vi "GSI-HVSwitch2.i attribute.vi"(0 "VI Refnum":refnum<vi>, 2 "CLASS.i attribute":T1={"SDEX VISA Cluster"={"VISA resource name"="", "HEX address"=0, "VISA Timeout Value (1000 ms)"=1000, "Lock Timeout (1000 ms)"=1000, "semaphore"=refnum, "Baud rate"=0, "revision"=enum."unknown", "deviceInfo"=""}, "SetVoltage SW0"=0.0, "SetVoltage SW1"=0.0, "ActTempAmp"=0.0, "ActTempPS1"=0.0, "ActTempPS2"=0.0, "mode"=enum."unknown", "interfaceInitialized"=FALSE, "serviceIDs"={"nomVoltage0ID"=0, "nomVoltage1ID"=0, "actTempAmpID"=0, "actTempPS1ID"=0, "actTempPS2ID"=0, "modeID"=0}, "usedChannels"=0} {"SDEX VISA Cluster"."HEX address" format="%.0x"}, 3 "Action":T6(ring), 5 "error in (no error)":errorcluster) -> (14 "VI Refnum out":refnum<vi>, 16 "CLASS.i attribute out":T1={"SDEX VISA Cluster"={"VISA resource name"="", "HEX address"=0, "VISA Timeout Value (1000 ms)"=1000, "Lock Timeout (1000 ms)"=1000, "semaphore"=refnum, "Baud rate"=0, "revision"=enum."unknown", "deviceInfo"=""}, "SetVoltage SW0"=0.0, "SetVoltage SW1"=0.0, "ActTempAmp"=0.0, "ActTempPS1"=0.0, "ActTempPS2"=0.0, "mode"=enum."unknown", "interfaceInitialized"=FALSE, "serviceIDs"={"nomVoltage0ID"=0, "nomVoltage1ID"=0, "actTempAmpID"=0, "actTempPS1ID"=0, "actTempPS2ID"=0, "modeID"=0}, "usedChannels"=0} {"SDEX VISA Cluster"."HEX address" format="%.0x"}, 19 "error out":errorcluster)   [LabVIEW 2014, in "GSI-HVSwitch2.lvlib"]
doc: "This is a so-called functional global variable. It manages the access to a global variable in a thread-safe way. \n\nHere the attribute data of all instances of THIS class are stored. This is done for performance reasons.\n\nLicense Agreement for this software:\n\nCopyright (C)\nGesellschaft für Schwerionenforschung, GSI\nPlanckstr. 1\n64291 Darmstadt\nGermany\n\nContact: D.Beck@gsi.de \n\nThis program is free software; you can redistribute it and/or modify it under the terms of the GNU General Public License as published by the Free Software Foundation; either version 2 of the license, or (at your option) any later version.\n\nThis program is distributed in the hope that it will be useful, but WITHOUT ANY WARRANTY; without even the implied warranty of MERCHANTABILITY or FITNESS FOR A PARTICULAR PURPOSE. See the GNU General License for more details (http://www.gnu.org).\n\nGesellschaft für Schwerionenforschung, GSI\nPlanckstr. 1, 64291 Darmstadt, Germany\nFor all questions and ideas contact: M.Richter@gsi.de, H.Brand@gsi.de or D.Beck@gsi.de.\nLast update: 17-JUN-2004"
uses:
  GSI-HVSwitch2.lvlib
  GSI-HVSwitch2.i attribute.ctl
  instr.lib/SDEX/SDEX.VISA Control.ctl
  instr.lib/SDEX/SDEX.revisionType.ctl
  GSI-HVSwitch2.mode.ctl
  CS_Core/CSSystem/CoreDefs/CoreDefs.error_type.ctl
  CS_Core/CSSystem/CoreLib/CoreLib.lvlib
  instr.lib/SDEX/SDEXDriver.lvlib
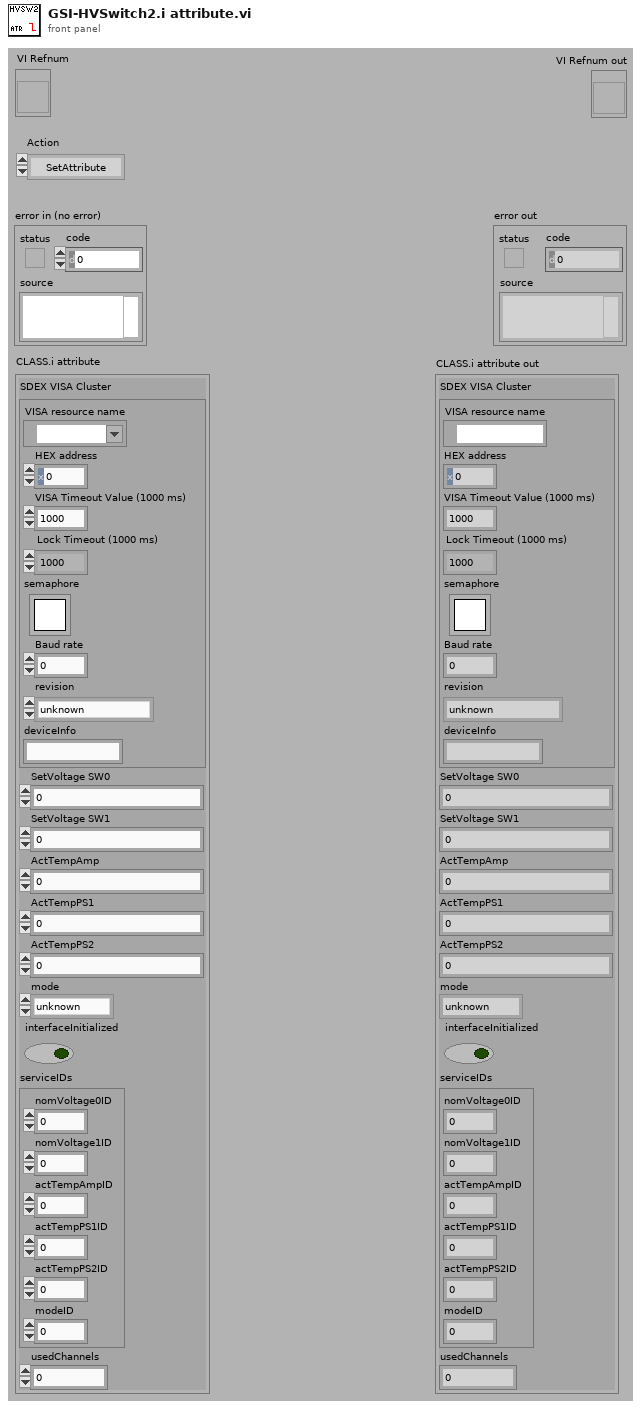
[diagram p1: front panel]
types:
  T1 = typedef "GSI-HVSwitch2.lvlib/GSI-HVSwitch2.i attribute.ctl" = cluster{"SDEX VISA Cluster":T2, "SetVoltage SW0":dbl, "SetVoltage SW1":dbl, "ActTempAmp":dbl, "ActTempPS1":dbl, "ActTempPS2":dbl, "mode":T5, "interfaceInitialized":bool, "serviceIDs":cluster{"nomVoltage0ID":i32, "nomVoltage1ID":i32, "actTempAmpID":i32, "actTempPS1ID":i32, "actTempPS2ID":i32, "modeID":i32}, "usedChannels":i32}
  T2 = typedef "SDEXDriver.lvlib/SDEX.VISA Control.ctl" = cluster{"VISA resource name":refnum<visa-resource-name>, "HEX address":u16, "VISA Timeout Value (1000 ms)":u32, "Lock Timeout (1000 ms)":u32, "semaphore":T3, "Baud rate":u32, "revision":T4, "deviceInfo":string}
  T3 = typedef "Semaphore RefNum" = refnum<k1>
  T4 = typedef "SDEXDriver.lvlib/SDEX.revisionType.ctl" = enum16{"unknown", "hvamp3", "hvswi1", "htrp0", "WDG0"}
  T5 = typedef "GSI-HVSwitch2.lvlib/GSI-HVSwitch2.mode.ctl" = enum16{"unknown", "switch", "stepper"}
  T6 = enum16{"SetAttribute", "GetAttribute", "CreateAttribute", "DestroyAttribute", "DestroyAllAtributes"}
  T7 = typedef "CoreDefs.error_type.ctl" = enum16{"no error", "can't load process", "can't unload process", "process does not exist", "can't install process", "can't remove process", "unknown function", "time out", "can't execute function", "duplicate queue name", "super not found", "caller queue invalid", "can't ping process", "unknown error", "VISA Error", "VISA timeout", "GPIB timeout", "GPIB error", "communication error", "data type mismatch", "can't read data from OPC server", "can't write data to OPC server", "OET error", "function not implemented", "process already exists", "invalid Shared Variable name", "error writing Shared Variable", "error reading Shared Variable", "invalid client name", "corrupt database", "unknown class", "call not authorized", "parameter out of range", "OET timeout: can't get data to modify", "invalid queue name", "requested operation incompatible with current state", "event undefined", "event disabled", "state undefined", "caller is not a friend", "EventBuilder: bad eventID", "EventBuilder: no DAQ devices", "a thread must not stop itself", "UNUSED ELEMENT4", "DiscArchiver: eventData incomplete", "DiscArchiver: eventData does not belong to run", "DiscArchiver: can't open file", "DiscArchiver: can't write to file", "DiscArchiver: available disc space low", "can't acquire semaphore", "error reading data from database", "notifier object is not existing", "can't register process", "can't unregister process", "illegal event type", "object disabled", "object already exists", "can't change state", "Instrument not found", "no connection to remote node", "invalid reference", "N/A", "UNUSED ELEMENT 1", "element not found", "illegal TCP/IP connection detected", "object does not exist", "invalid access ID", "unknown CS system", "invalid privilige", "unsupported data type", "unsupported server type", "IO server already exists", "Shared Variable already exists"}
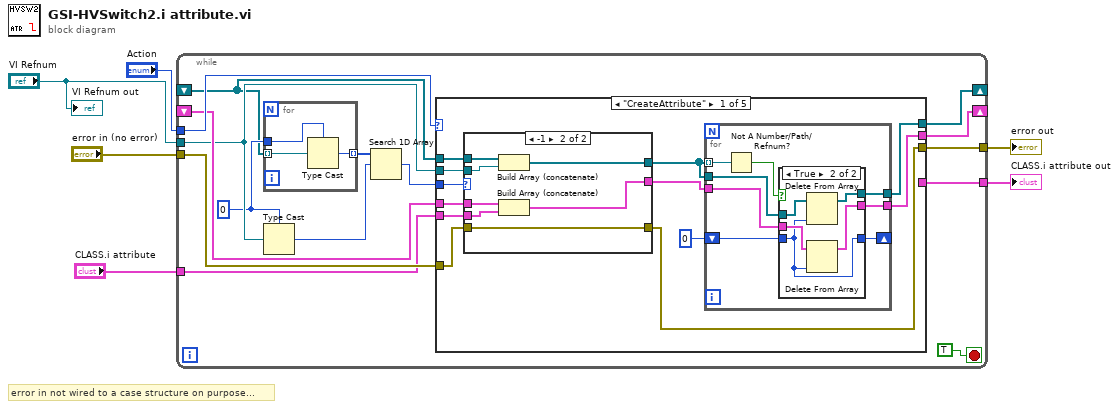
[diagram p0: block diagram]
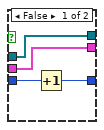
[diagram p2: hidden frame]
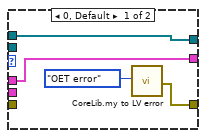
[diagram p3: hidden frame]
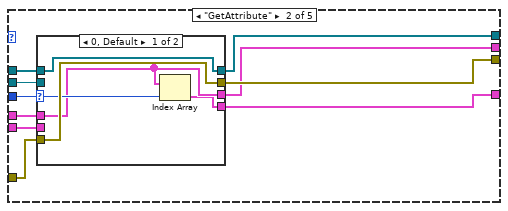
[diagram p4: hidden frame]
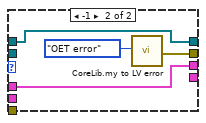
[diagram p5: hidden frame]
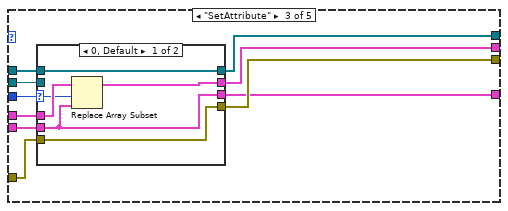
[diagram p6: hidden frame]
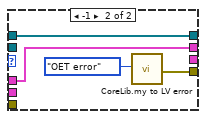
[diagram p7: hidden frame]
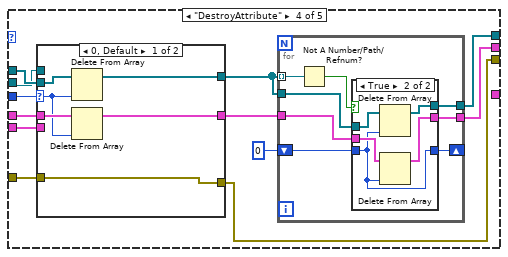
[diagram p8: hidden frame]
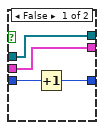
[diagram p9: hidden frame]
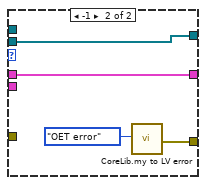
[diagram p10: hidden frame]
diagram:
  # "error in not wired to a case structure on purpose..."
  n1 = while {
    shift-right: [w15] -> _
    shift-left: _ -> [w16]
    tunnel: "Action" -> [w20]
    shift-right: [w17] -> _
    shift-left: _ -> [w7]
    tunnel: "error in (no error)" -> [w19]
    tunnel: [w18] -> w4
    tunnel: "CLASS.i attribute" -> [w14]
    tunnel: [w12] -> w2
    tunnel: "VI Refnum" -> [w10]
    stop <- TRUE stop-if-true
    w9 = 0
    n2 = for {
      tunnel: w9 -> [w24]
      tunnel: [w23] -> w8 mode=indexing
      tunnel: w7 -> [w22] mode=indexing
      n3 = Type Cast(type=w24, x=w22) -> (*(type *) &x=w23:i32)
    }
    n4 = Type Cast(type=w9, x=w10) -> (*(type *) &x=w11:i32)
    n5 = Search 1D Array(1D array=w8, element=w11) -> (index of element=w13:i32)  [unwired: 1 in]
    n6 = case shown="\"CreateAttribute\"" w20 {
      tunnel: w7 -> [w34 w72 w91 w113 _]
      tunnel: w10 -> [w33 w70 w89 w112 _]
      tunnel: w19 -> [w36 w74 w93 w115 w143]
      tunnel: [w35 w73 w92 w114 w143] -> w18
      tunnel: [w28 w71 w90 w107 _] -> w17
      tunnel: w16 -> [w32 w69 w88 w111 _]
      tunnel: [w27 w68 w87 w106 _] -> w15
      tunnel: w14 -> [w31 w67 w86 w110 _]
      tunnel: w13 -> [w30 w66 w85 w109 _]
      tunnel: [_ w65 w84 _ _] -> w12
      frame "CreateAttribute" {
        n7 = case shown="-1" w30 {
          tunnel: w36 -> [_ w64]
          tunnel: [w56 w64] -> w35
          tunnel: w34 -> [w55 w63]
          tunnel: [w55 w62] -> w25
          tunnel: w33 -> [_ w61]
          tunnel: w32 -> [w54 w60]
          tunnel: [w54 w59] -> w26
          tunnel: w31 -> [_ w58]
          frame 0, Default {
            n8 = call "CoreLib.my to LV error.vi"("ErrorTypes"=CoreDefs.error_type."OET error") -> ("myErrorCluster"=w56:errorcluster)  [unwired: 17 in, 1 out]
          }
          frame -1 {
            n9 = Build Array (concatenate)(w63, w61) -> (w62:refnum<vi>[])
            n10 = Build Array (concatenate)(w60, w58) -> (w59:T1[])
          }
        }
        n11 = for {
          tunnel: w25 -> [w41]
          tunnel: [w40] -> w28
          tunnel: [w44] -> w27
          tunnel: w26 -> [w43]
          tunnel: w25 -> [w39] mode=indexing
          shift-right: [w38] -> _
          shift-left: 0 -> [w37]
          n12 = Not A Number/Path/Refnum?(number/path/refnum=w39) -> (NaN/Path/Refnum?=w42:bool)
          n13 = case shown="True" w42 {
            tunnel: [w48 w53] -> w44
            tunnel: w43 -> [w48 w52]
            tunnel: [w47 w50] -> w40
            tunnel: w41 -> [w47 w51]
            tunnel: w37 -> [w46 w49]
            tunnel: [w45 w49] -> w38
            frame False {
              n14 = Increment(x=w46) -> (x+1=w45:i32)
            }
            frame True {
              n15 = Delete From Array(array=w51, index=w49) -> (array with subset deleted=w50:refnum<vi>[])  [unwired: 1 in, 1 out]
              n16 = Delete From Array(array=w52, index=w49) -> (array with subset deleted=w53:T1[])  [unwired: 1 in, 1 out]
            }
          }
        }
      }
      frame "GetAttribute" {
        n17 = case shown="0, Default" w66 {
          selector: w66 -> [w77 _]
          tunnel: w74 -> [w79 _]
          tunnel: [w79 w82] -> w73
          tunnel: w72 -> [w78 w81]
          tunnel: [w78 w81] -> w71
          tunnel: w70 -> [_ _]
          tunnel: w69 -> [w76 w80]
          tunnel: [w76 w80] -> w68
          tunnel: w67 -> [_ _]
          tunnel: [w75 _] -> w65
          frame 0, Default {
            n18 = Index Array(array=w76, index=w77) -> (element=w75:T1)
          }
          frame -1 {
            n19 = call "CoreLib.my to LV error.vi"("ErrorTypes"=CoreDefs.error_type."OET error") -> ("myErrorCluster"=w82:errorcluster)  [unwired: 17 in, 1 out]
          }
        }
      }
      frame "SetAttribute" {
        n20 = case shown="0, Default" w85 {
          selector: w85 -> [w95 _]
          tunnel: w93 -> [w99 _]
          tunnel: [w99 w102] -> w92
          tunnel: w91 -> [w98 w101]
          tunnel: [w98 w101] -> w90
          tunnel: w89 -> [_ _]
          tunnel: w88 -> [w97 w100]
          tunnel: [w96 w100] -> w87
          tunnel: w86 -> [w94 _]
          tunnel: [w94 _] -> w84
          frame 0, Default {
            n21 = Replace Array Subset(array=w97, new element=w94, index=w95) -> (w96:T1[])
          }
          frame -1 {
            n22 = call "CoreLib.my to LV error.vi"("ErrorTypes"=CoreDefs.error_type."OET error") -> ("myErrorCluster"=w102:errorcluster)  [unwired: 17 in, 1 out]
          }
        }
      }
      frame "DestroyAttribute" {
        n23 = case shown="0, Default" w109 {
          selector: w109 -> [w134 _]
          tunnel: w115 -> [w138 _]
          tunnel: [w138 w141] -> w114
          tunnel: w113 -> [w137 w140]
          tunnel: [w136 w140] -> w104
          tunnel: w112 -> [_ _]
          tunnel: w111 -> [w135 w139]
          tunnel: [w133 w139] -> w105
          tunnel: w110 -> [_ _]
          frame 0, Default {
            n24 = Delete From Array(array=w137, index=w134) -> (array with subset deleted=w136:refnum<vi>[])  [unwired: 1 in, 1 out]
            n25 = Delete From Array(array=w135, index=w134) -> (array with subset deleted=w133:T1[])  [unwired: 1 in, 1 out]
          }
          frame -1 {
            n26 = call "CoreLib.my to LV error.vi"("ErrorTypes"=CoreDefs.error_type."OET error") -> ("myErrorCluster"=w141:errorcluster)  [unwired: 17 in, 1 out]
          }
        }
        n27 = for {
          tunnel: w104 -> [w120]
          tunnel: [w119] -> w107
          tunnel: [w123] -> w106
          tunnel: w105 -> [w122]
          tunnel: w104 -> [w118] mode=indexing
          shift-right: [w117] -> _
          shift-left: 0 -> [w116]
          n28 = Not A Number/Path/Refnum?(number/path/refnum=w118) -> (NaN/Path/Refnum?=w121:bool)
          n29 = case shown="True" w121 {
            tunnel: [w127 w132] -> w123
            tunnel: w122 -> [w127 w131]
            tunnel: [w126 w129] -> w119
            tunnel: w120 -> [w126 w130]
            tunnel: w116 -> [w125 w128]
            tunnel: [w124 w128] -> w117
            frame False {
              n30 = Increment(x=w125) -> (x+1=w124:i32)
            }
            frame True {
              n31 = Delete From Array(array=w130, index=w128) -> (array with subset deleted=w129:refnum<vi>[])  [unwired: 1 in, 1 out]
              n32 = Delete From Array(array=w131, index=w128) -> (array with subset deleted=w132:T1[])  [unwired: 1 in, 1 out]
            }
          }
        }
      }
      frame "DestroyAllAtributes" {
      }
    }
  }
  "error out" <- w4
  "CLASS.i attribute out" <- w2
  "VI Refnum out" <- "VI Refnum"
